vi "Coord window-Save load coordinates file.vi"(8 "error in (no error)":errorcluster, 9 "Function":T1) -> (0 "error out":errorcluster)   [LabVIEW 2013]
uses:
  Visualisation/Functional Imaging Viewer/SubVIs/Experiment header interface/Typedefs/Save-Load-Save as-Load last enum.ctl
  Globals/Coord window-Globals.vi
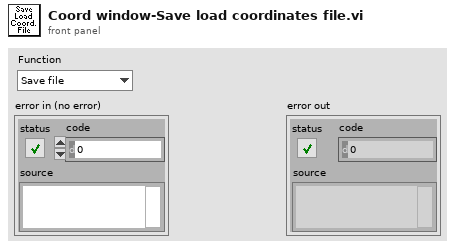
[diagram p1: front panel]
types:
  T1 = typedef "Save-Load-Save as-Load last enum.ctl" = enum16{"Save file", "Save file as", "Load file", "Load last file"}
  T2 = typedef "Coordinate list window refs.ctl" = cluster{"Window Name (i.e. Key)":string, "menu reference":refnum<k9>, "VI's reference":refnum<vi>, "Pane 1":refnum<vi>, "Pane 2":refnum<vi>, "Coord Listbox":refnum<vi>, "File name":refnum<vi>, "Picture Map":refnum<vi>, "Stage XYZ Position ind.":refnum<vi>}
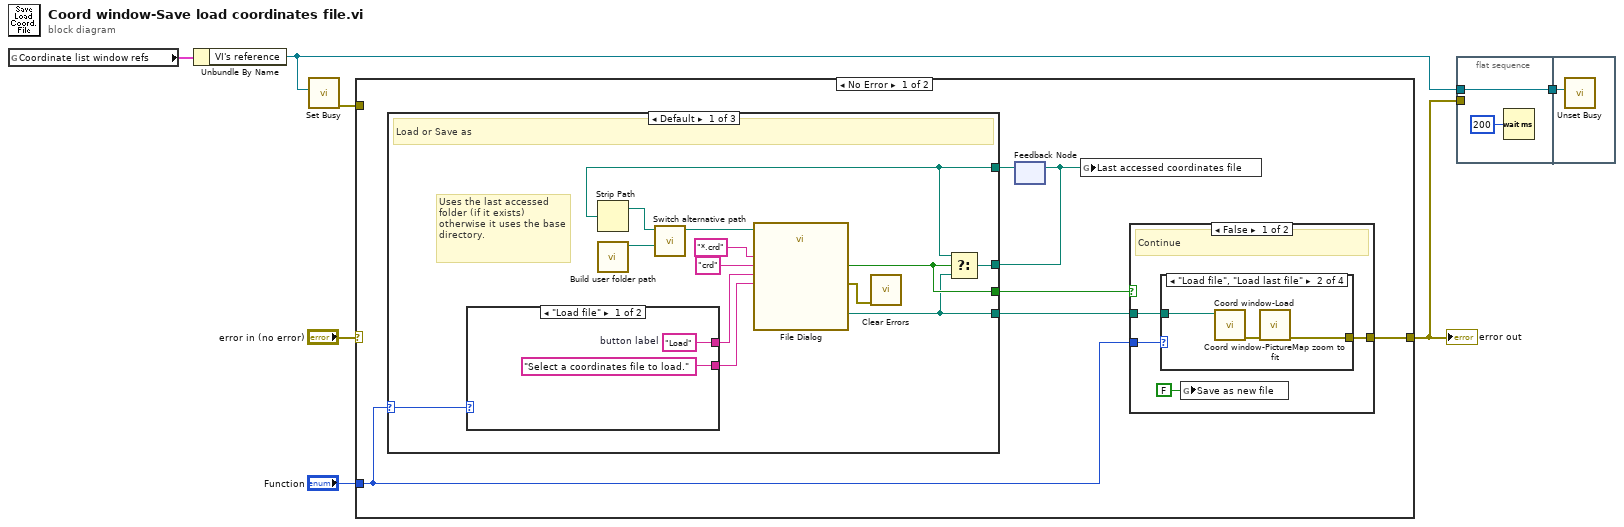
[diagram p0: block diagram]
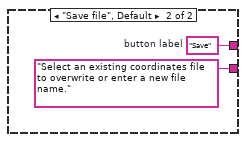
[diagram p2: hidden frame]
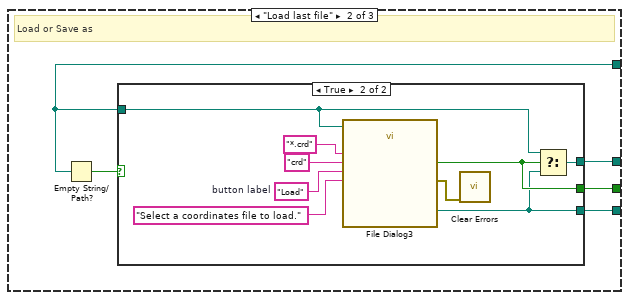
[diagram p3: hidden frame]
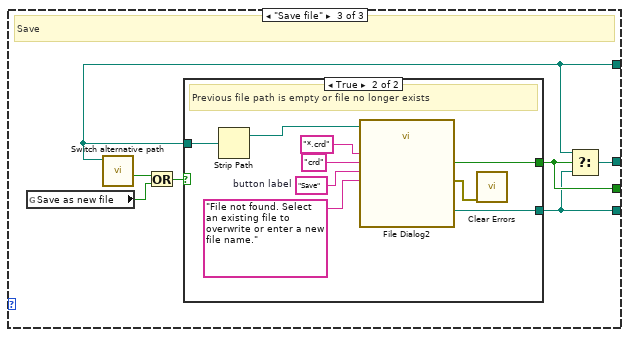
[diagram p5: hidden frame]
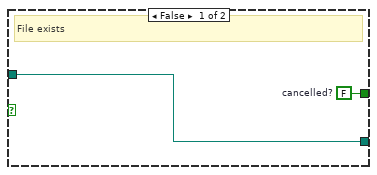
[diagram p6: hidden frame]
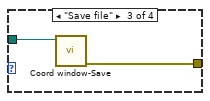
[diagram p8: hidden frame]
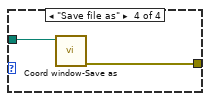
[diagram p9: hidden frame]
diagram:
  n1 = global read "Coord window-Globals.vi" "Coordinate list window refs"() -> (w5:T2)
  n2 = Unbundle By Name(w5) -> ("VI's reference"=w3:refnum<vi>)
  n3 = call <vilib>:"Set Busy.vi"("VI reference (current VI)"=w3) -> ("error out"=w4:errorcluster)  [unwired: 9 in, 1 out]
  n4 = case shown="No Error" "error in (no error)" {
    selector: "error in (no error)" -> [_ w75]
    tunnel: "Function" -> [w8 _]
    tunnel: [w10 w75] -> w2
    tunnel: w4 -> [_ _]
    frame No Error {
      n5 = feedback #1() -> (w13:path)  [unwired: 1 in]
      n6 = case shown="Default" w8 {
        selector: w8 -> [w17 _ _]
        tunnel: [w22 w35 w52] -> w9
        tunnel: w13 -> [w16 w32 w49]
        tunnel: [w19 w34 w51] -> w12
        tunnel: [w18 w33 w50] -> w11
        frame Default {
          # "Uses the last accessed folder (if it exists) otherwise it uses the base directory."
          # "Load or Save as"
          n7 = case shown="\"Load file\"" w17 {
            tunnel: [w28 w30] -> w24
            tunnel: ["Select a coordinates file to load." ("prompt") "Select an existing coordinates file to overwrite or enter a new file name." ("prompt")] -> w21
            frame "Load file" {
              w28 = "Load"  # button label
            }
            frame "Save file", Default {
              w30 = "Save"  # button label
            }
          }
          n8 = Strip Path(path=w16) -> (stripped path=w15:path)  [unwired: 1 out]
          n9 = call "Build user folder path.vi"() -> ("Daily folder path with user folder appended?"=w14:path)  [unwired: 11 in]
          n10 = call "Switch alternative path.vi"("Alternative path"=w14, "Original path"=w15) -> ("Output path"=w23:path)  [unwired: 7 in, 2 out]
          n11 = call "File Dialog"("start path"=w23, "prompt"=w21, "button label"=w24, "pattern (all files)"="*.crd", "pattern label"="crd") -> ("selected path"=w18:path, "cancelled"=w19:bool, "error out"=w26:errorcluster)  [unwired: 7 in, 1 out]
          n12 = call <vilib>:"Clear Errors.vi"("error in (no error)"=w26) -> ()  [unwired: 6 in, 1 out]
          n13 = Select(t=w16, s=w19, f=w18) -> (s? t:f=w22:path)
        }
        frame "Load last file" {
          # "Load or Save as"
          n14 = Empty String/Path?(string/path=w32) -> (empty?=w31:bool)
          n15 = case shown="True" w31 {
            tunnel: [w36 w42] -> w35
            tunnel: [_ w39] -> w34
            tunnel: [w36 w38] -> w33
            tunnel: w32 -> [w36 w37]
            frame False {
            }
            frame True {
              w43 = "Load"  # button label
              n16 = call "File Dialog3"("start path"=w37, "prompt"="Select a coordinates file to load.", "button label"=w43, "pattern (all files)"="*.crd", "pattern label"="crd") -> ("selected path"=w38:path, "cancelled"=w39:bool, "error out"=w45:errorcluster)  [unwired: 7 in, 1 out]
              n17 = call <vilib>:"Clear Errors.vi"("error in (no error)"=w45) -> ()  [unwired: 6 in, 1 out]
              n18 = Select(t=w37, s=w39, f=w38) -> (s? t:f=w42:path)
            }
          }
        }
        frame "Save file" {
          # "Save"
          n19 = global read "Coord window-Globals.vi" "Save as new file"() -> (w46:bool)
          n20 = call "Switch alternative path.vi"("Original path"=w49) -> ("Path is empty or does not exist"=w48:bool)  [unwired: 8 in, 2 out]
          n21 = Or(x=w48, y=w46) -> (x .or. y?=w47:bool)
          n22 = case shown="True" w47 {
            tunnel: [w54 w58] -> w51
            tunnel: [w53 w57] -> w50
            tunnel: w49 -> [w53 w56]
            frame False {
              w54 = FALSE  # cancelled?
              # "File exists"
            }
            frame True {
              w61 = "Save"  # button label
              # "Previous file path is empty or file no longer exists"
              n23 = Strip Path(path=w56) -> (stripped path=w55:path)  [unwired: 1 out]
              n24 = call "File Dialog2"("start path"=w55, "prompt"="File not found. Select an existing file to overwrite or enter a new file name.", "button label"=w61, "pattern (all files)"="*.crd", "pattern label"="crd") -> ("selected path"=w57:path, "cancelled"=w58:bool, "error out"=w63:errorcluster)  [unwired: 7 in, 1 out]
              n25 = call <vilib>:"Clear Errors.vi"("error in (no error)"=w63) -> ()  [unwired: 6 in, 1 out]
            }
          }
          n26 = Select(t=w49, s=w51, f=w50) -> (s? t:f=w52:path)
        }
      }
      n27 = feedback-in #1(w9) -> ()
      n28 = global write "Coord window-Globals.vi" "Last accessed coordinates file"(w9) -> ()
      n29 = case shown="False" w12 {
        tunnel: w8 -> [w67 _]
        tunnel: w11 -> [w66 _]
        tunnel: [w65 _] -> w10
        frame False {
          # "Continue"
          n30 = case shown="\"Load file\", \"Load last file\"" w67 {
            tunnel: w66 -> [_ w70 w71 w73]
            tunnel: [_ w68 w72 w74] -> w65
            frame Default {
            }
            frame "Load file", "Load last file" {
              n31 = call "Coord window-Load.vi"("selected path"=w70) -> ("error out"=w69:errorcluster)  [unwired: 10 in]
              n32 = call "Coord window-PictureMap zoom to fit.vi"("error in"=w69) -> ("error out"=w68:errorcluster)  [unwired: 10 in]
            }
            frame "Save file" {
              n33 = call "Coord window-Save.vi"("file path"=w71) -> ("error out"=w72:errorcluster)  [unwired: 10 in]
            }
            frame "Save file as" {
              n34 = call "Coord window-Save as.vi"("file path"=w73) -> ("error out"=w74:errorcluster)  [unwired: 10 in]
            }
          }
          n35 = global write "Coord window-Globals.vi" "Save as new file"(FALSE ("Save as new file")) -> ()
        }
        frame True {
          # "Cancelled"
        }
      }
    }
    frame Error {
    }
  }
  "error out" <- w2
  n36 = flat-sequence {
    tunnel: w2 -> [_]
    tunnel: w3 -> [w77]
    tunnel: [w77] -> w1
    tunnel: w1 -> [w78]
    frame #0 {
      n37 = Wait (ms)(milliseconds to wait=u32 200) -> ()  [unwired: 1 out]
    }
    frame #1 {
      n38 = call <vilib>:"Unset Busy.vi"("VI reference (current VI)"=w78) -> ()  [unwired: 10 in, 1 out]
    }
  }
